vi "Delay PanelUpdata.vi"(8 "error in":errorcluster caption="错误输入（无错误）", 10 "延迟前面板更新":bool, 11 "PanelRootNode 输入":refnum<class "PanelRootNode.lvclass"> caption="DNL_LabVIEW Object in") -> (0 "error out":errorcluster caption="错误输出", 3 "PanelRootNode 输出":refnum<class "PanelRootNode.lvclass"> caption="DNL_LabVIEW Object out")   [LabVIEW 2016, in "PanelRootNode.lvclass"]
uses:
  PanelRootNode.lvclass
  PanelRootNode.lvclass/PanelRootNode.ctl
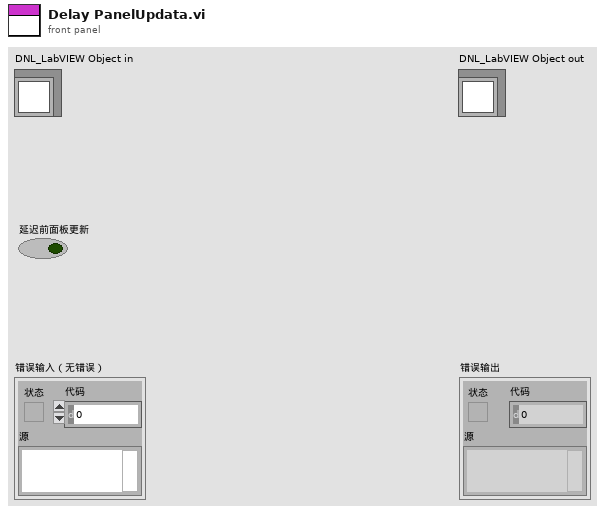
[diagram p1: front panel]
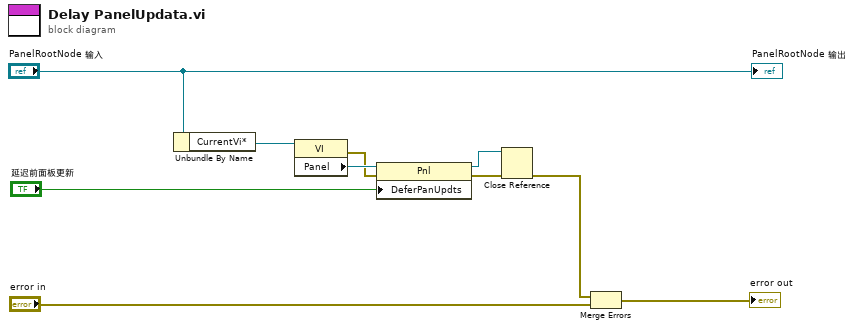
[diagram p0: block diagram]
diagram:
  n1 = Unbundle By Name("PanelRootNode 输入") -> ("CurrentVi*"=w8:refnum<vi>)
  n2 = property class="VI"(reference=w8) -> (error out=w6:errorcluster, "Panel"=w7:refnum<vi>)  [unwired: 1 in, 1 out]
  n3 = property class="Pnl"(reference=w7, error in=w6, "DeferPanUpdts"="延迟前面板更新") -> (reference out=w4:refnum<vi>, error out=w5:errorcluster)
  n4 = Close Reference(reference=w4, error in (no error)=w5) -> (error out=w3:errorcluster)
  n5 = Merge Errors(w3, "error in") -> (→"error out":errorcluster)
  "PanelRootNode 输出" <- "PanelRootNode 输入"
